vi "a.vi"(6 "string":string, 8 "TAGs 2":string[](array[string]), 10 "string 4":string[][](array[string]), 11 "string 3":string[](array[string])) -> ()   [LabVIEW 2015]
panel:
  in  "number 2":i32[](array[numeric])
  in  "number 3":i32
  in  "number":i32
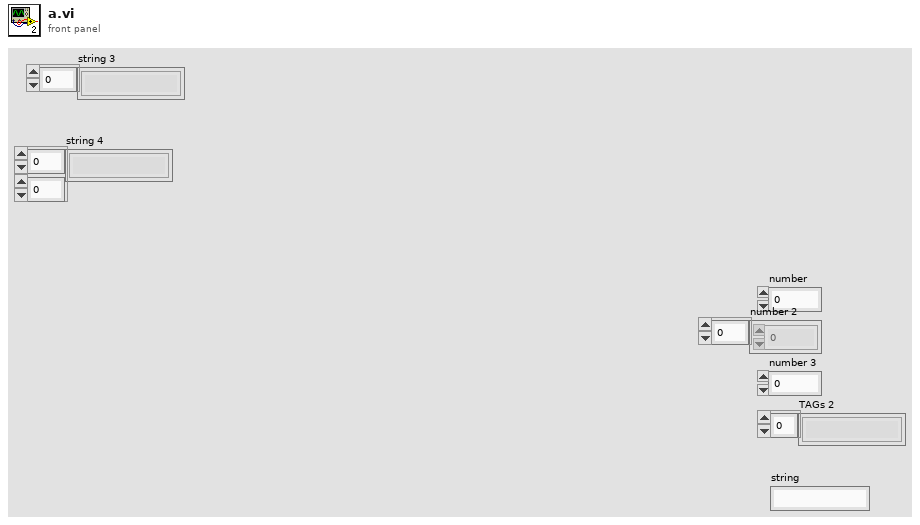
[diagram p1: front panel]
types:
  T1 = enum16{"open", "replace", "create", "open or create", "replace or create", "replace or create with confirmation"}
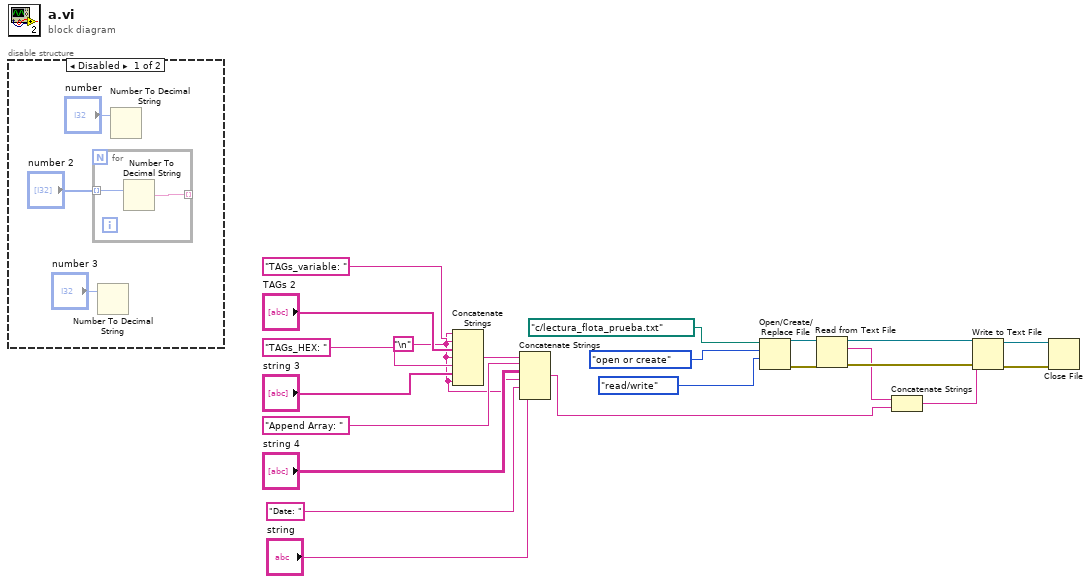
[diagram p0: block diagram]
diagram:
  w3 = "\n"
  n1 = disable-structure shown="Disabled" {
    frame Disabled {
      n2 = for {
        tunnel: [w27] -> _ mode=indexing
        tunnel: "number 2" -> [w26] mode=indexing
        n3 = Number To Decimal String(number=w26) -> (decimal integer string=w27:string)  [unwired: 1 in]
      }
      n4 = Number To Decimal String(number="number 3") -> ()  [unwired: 1 in, 1 out]
      n5 = Number To Decimal String(number="number") -> ()  [unwired: 1 in, 1 out]
    }
    frame Enabled {
    }
  }
  n6 = Concatenate Strings(w3, "TAGs_variable: " ("string"), "TAGs 2", w3, "TAGs_HEX: " ("string"), "string 3", w3) -> (w11:string)
  n7 = Concatenate Strings(w11, "Append Array: " ("string"), "string 4", w3, "Date: " ("string"), "string") -> (w10:string)
  n8 = Open/Create/Replace File(file path (use dialog)=path "c:/lectura_flota_prueba.txt", operation (0:open)=T1."open or create", access (0:read/write)=enum16{"read/write", "read-only", "write-only"}."read/write") -> (refnum out=w15:refnum<file>, error out=w17:errorcluster)  [unwired: 3 in, 1 out]
  n9 = Read from Text File(file (use dialog)=w15, error in=w17) -> (refnum out=w14:refnum<file>, text=w13:string, error out=w16:errorcluster)  [unwired: 2 in, 1 out]
  n10 = Concatenate Strings(w13, w10) -> (w12:string)
  n11 = Write to Text File(file (use dialog)=w14, text=w12, error in=w16) -> (refnum out=w21:refnum<file>, error out=w22:errorcluster)  [unwired: 1 in, 1 out]
  n12 = Close File(refnum=w21, error in=w22) -> ()  [unwired: 2 out]
